vi "Unrecoverable Writer Error.vi"() -> ()   [LabVIEW 2018]
uses:
  api/Failure Information.ctl
  api/Log Record.ctl
  api/logger_class/Internal Log Levels.ctl
  api/Log Levels.ctl
  api/configuration/handlers/file_handler/File Handler.lvclass
  C:/Users/Colin/Documents/software_projects/glog/src/api/extension/formatting_handler_interface/Formatting Handler.lvclass
  custom_classes/test_handler/Test Handler.lvclass
  api/logger_class/Logger.lvclass
  api/GLog.lvlib
panel:
  out "failure info":T1 {"Log Record"."timestamp" format="%<%x %.3X>T"}
  out "error out":errorcluster
  # "Locals"
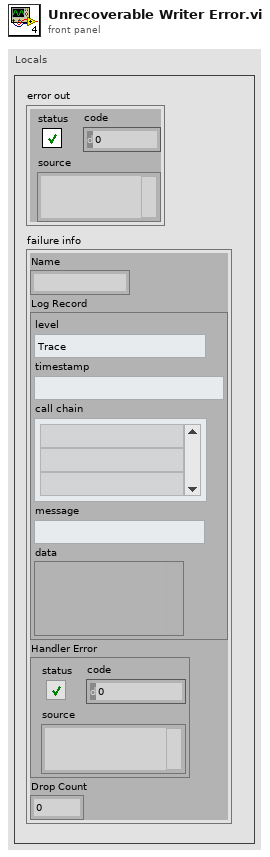
[diagram p1: front panel]
types:
  T1 = typedef "GLog.lvlib/Failure Information.ctl" = cluster{"Name":string, "Log Record":T2, "Handler Error":errorcluster, "Drop Count":u32}
  T2 = typedef "GLog.lvlib/Log Record.ctl" = cluster{"level":T3, "timestamp":timestamp, "call chain":string[], "message":string, "data":variant}
  T3 = typedef "GLog.lvlib/Internal Log Levels.ctl" = enum16{"Trace", "Debug", "Info", "Warning", "Error", "Critical", "Internal"}
  T4 = typedef "GLog.lvlib/Log Levels.ctl" = enum16{"Trace", "Debug", "Info", "Warning", "Error", "Critical"}
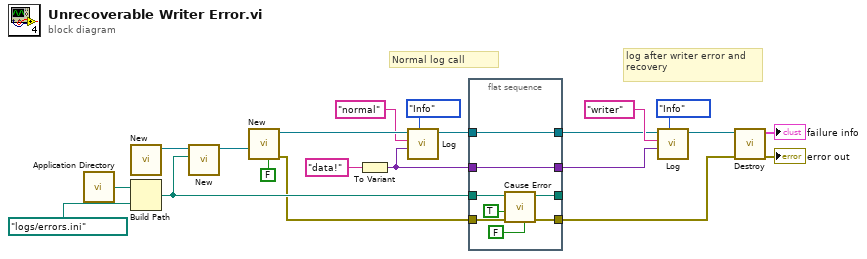
[diagram p0: block diagram]
diagram:
  # "log after writer error and recovery"
  # "Normal log call"
  n1 = call <vilib>:"Application Directory.vi"() -> ("Application Directory"=w7:path)
  n2 = call "New.vi"() -> ("file handler"=w21:refnum<class "File Handler.lvclass">)  [unwired: 11 in]
  n3 = Build Path(base path=w7, name or relative path=path "logs/errors.ini") -> (appended path=w13:path)
  n4 = call "New.vi"("config file"=w13, "subhandler"=w21) -> ("test handler out"=w20:refnum<class "Test Handler.lvclass">)  [unwired: 9 in]
  n5 = call "New.vi"("dialog on failure? (T)"=FALSE, "log handler (file handler)"=w20) -> ("error out"=w12:errorcluster, "logger"=w18:refnum<class "Logger.lvclass">)  [unwired: 8 in]
  n6 = To Variant(anything="data!" ("message")) -> (Variant=w4:variant)
  n7 = call "Log.vi"("log level"=Log_Levels."Info" ("level"), "data (null)"=w4, "message"="normal", "logger in"=w18) -> ("logger out"=w9:refnum<class "Logger.lvclass">)  [unwired: 7 in]
  n8 = flat-sequence {
    tunnel: w13 -> [w29]
    tunnel: w12 -> [w28]
    tunnel: [w27] -> w11
    tunnel: [w26] -> _
    tunnel: [w25] -> w10
    tunnel: w9 -> [w25]
    tunnel: [w24] -> w3
    tunnel: w4 -> [w24]
    frame #0 {
      n9 = call "Cause Error.vi"("writer recovery? (T)"=FALSE, "error in (no error)"=w28, "writer error? (F)"=TRUE ("formatter error? (F)"), "ini file path"=w29) -> ("error out"=w27:errorcluster, "ini file path"=w26:path)  [unwired: 6 in]
    }
  }
  n10 = call "Log.vi"("log level"=Log_Levels."Info" ("level"), "data (null)"=w3, "message"="writer", "logger in"=w10) -> ("logger out"=w8:refnum<class "Logger.lvclass">)  [unwired: 7 in]
  n11 = call "Destroy.vi"("error in (no error)"=w11, "logger in"=w8) -> ("error out"=→"error out":errorcluster, "failure info"=→"failure info":T1)  [unwired: 8 in]
